vi "NI XNET CAN Signal Logger - Executor.vi"(8 "error in (no error)":errorcluster, 11 "Executor Command":refnum<user-event>) -> (0 "error out":errorcluster)   [LabVIEW 2021, in "XNET-CAN-Signal-Logger.lvlib"]
uses:
  XNET-CAN-Signal-Logger.lvlib
  Typedef/Def-Executor Command.ctl
  Def-ExecutorConfigurations.ctl
  Typedef/Def-LogSpec.ctl
  Typedef/Def-CAN Port Configuration.ctl
  Typedef/Def-Data Queue Ref.ctl
  Typedef/Def-Data Queue Type.ctl
  <userlib>/_NEVSTOP/NEVSTOP_TimerEngine/_Typedef/Timer-UserEvent.ctl
  Typedef/Def-GSTOP.ctl
  SubVIs/Global Variables.vi
  <userlib>/_NEVSTOP/GlobalStop/_gStop.vi
  <userlib>/_NEVSTOP/GlobalStop/GSTOP.lvlib
  <userlib>/_NEVSTOP/NEVSTOP_TimerEngine/TimerEngine.lvclass
panel:
  out "Monitor.Values":variant[](array[variant])
  out "Monitor.Names":variant[](array[variant])
  out "Signal Data":waveform(dbl)[](array[waveform])
  out "Signal Names":string[](array[string])
  out "Debug.WriterState":bool
  out "Debug.ReadersState":bool[](array[boolean])
  out "State":string="Preview..." caption="State:"
  out "# elements in queue":i32 caption="# elements in queue:"
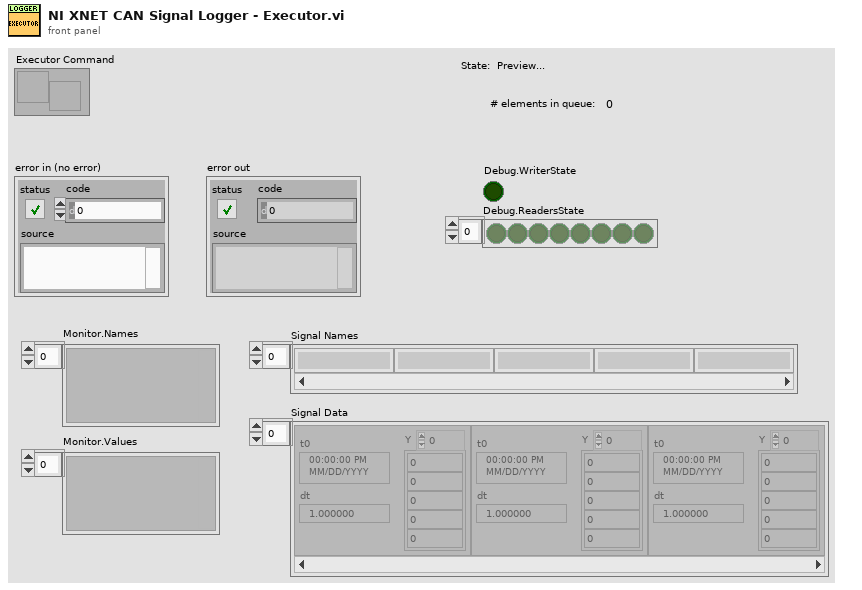
[diagram p1: front panel]
types:
  T1 = typedef "XNET-CAN-Signal-Logger.lvlib/Def-ExecutorConfigurations.ctl" = cluster{"LogSpec":T2, "CAN Configurations":T3[]}
  T2 = typedef "XNET-CAN-Signal-Logger.lvlib/Def-LogSpec.ctl" = cluster{"Log file folder":path, "Log file name":string, "Segment Files":bool, "Segment File Size":i64}
  T3 = typedef "XNET-CAN-Signal-Logger.lvlib/Def-CAN Port Configuration.ctl" = cluster{"CAN Interface":refnum<k21>, "XNET Cluster":refnum<k21>, "#Signals":i32, "Sample Rate (Hz)":dbl}
  T4 = enum32{"Invalid", "Standard", "Closed", "Hidden", "Minimized", "Maximized"}
  T5 = enum32{"invalid app kind", "Development System", "Run Time System", "Student Edition", "Embedded LabVIEW", "Evaluation", "Custom"}
  T6 = typedef "XNET-CAN-Signal-Logger.lvlib/Def-Executor Command.ctl" = cluster{"Command":string, "Data":variant}
  T7 = typedef "XNET-CAN-Signal-Logger.lvlib/Def-Data Queue Type.ctl" = cluster{"PackageID":i32, "Data":waveform(dbl)[]}
  T8 = typedef "XNET-CAN-Signal-Logger.lvlib/Def-GSTOP.ctl" = enum16{"Writer", "Readers"}
  T9 = typedef "XNET-CAN-Signal-Logger.lvlib/Def-Data Queue Ref.ctl" = refnum<queue>
  T10 = cluster{"Core":cluster{"Current VI Reference":refnum<vi>, "Close Panel on Exit?":bool}, "LogSpec":T2, "LogFilePath":path, "LogTS":timestamp, "CAN Configurations":T3[], "Signals to Monitor":string[][], "Data Queue Ref":T9, "Error Queue Ref":refnum<queue>, "State":string, "Executor Command":refnum<user-event>}
  T11 = cluster{"Current VI Reference":refnum<vi>, "Close Panel on Exit?":bool}
  T12 = typedef "TimerEngine.lvlib/TimerEngine.lvclass/Timer-UserEvent.ctl" = refnum<user-event>
  T13 = typedef "TimerEngine.lvlib/TimerEngine.lvclass/Timer-Userevent.ctl" = refnum<user-event>
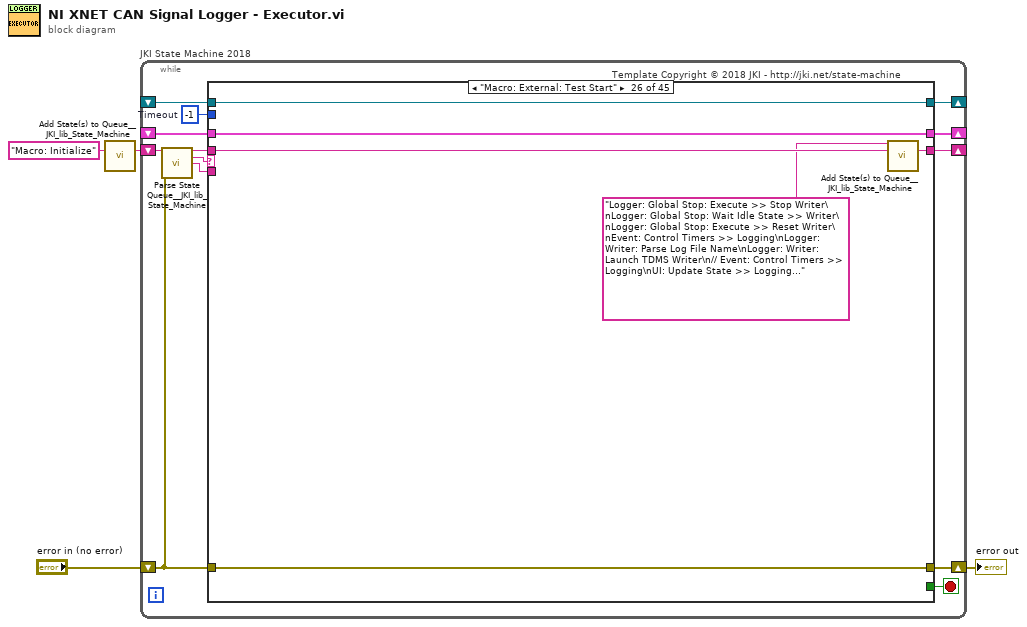
[diagram p0: block diagram]
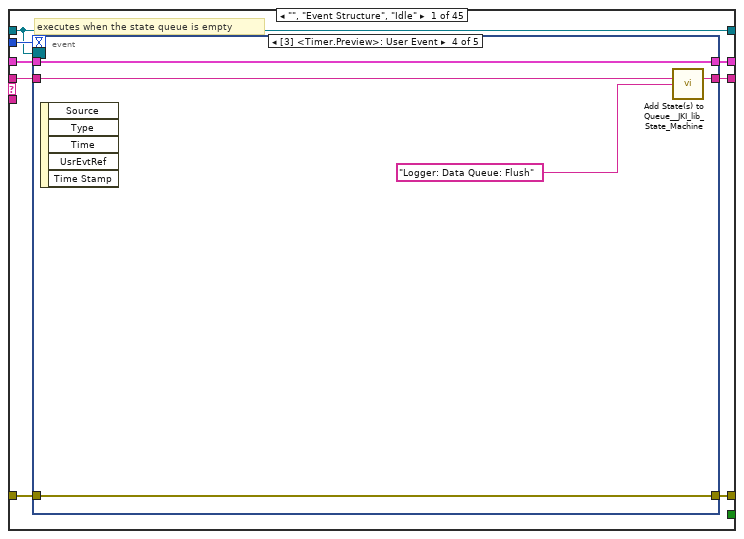
[diagram p2: hidden frame]
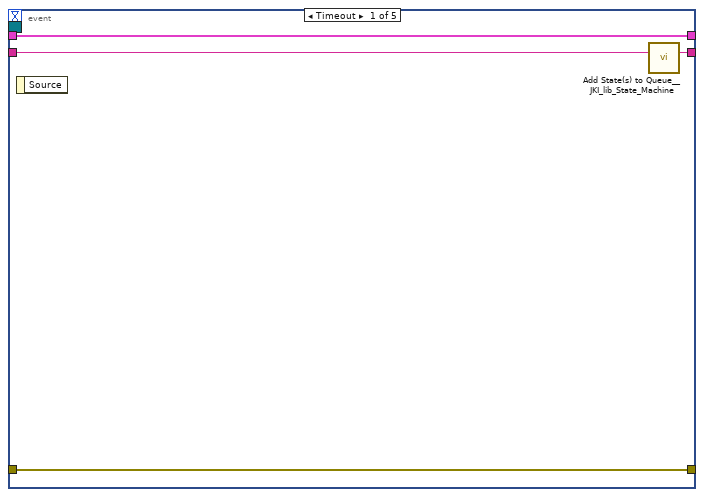
[diagram p3: hidden frame]
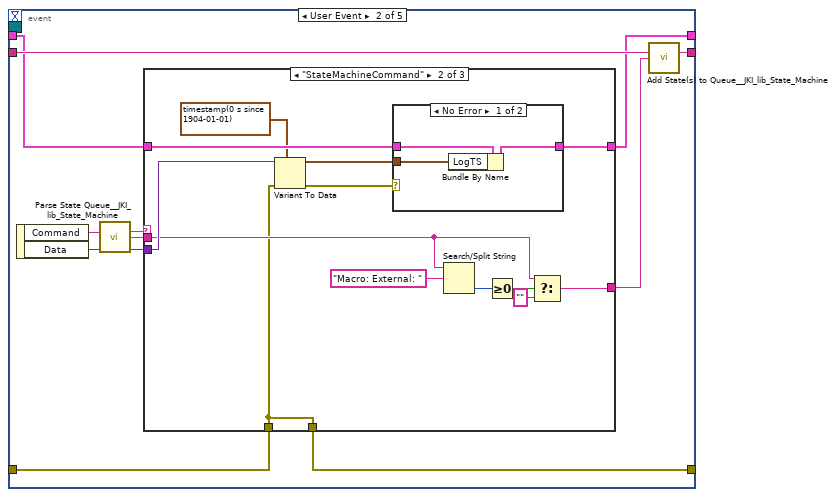
[diagram p4: hidden frame]
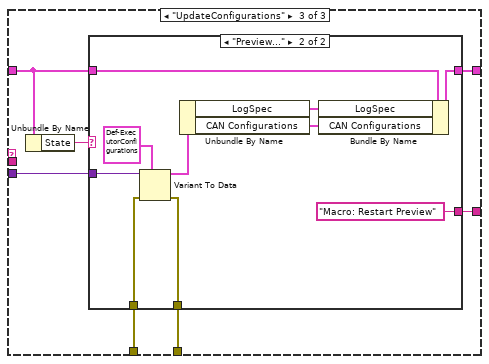
[diagram p7: hidden frame]
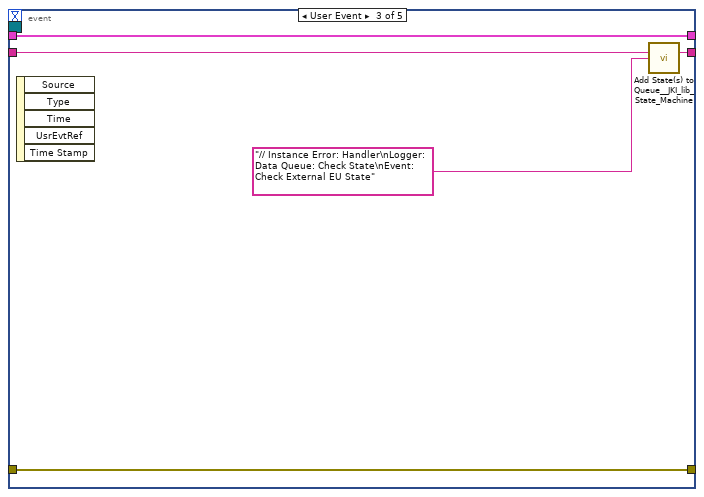
[diagram p9: hidden frame]
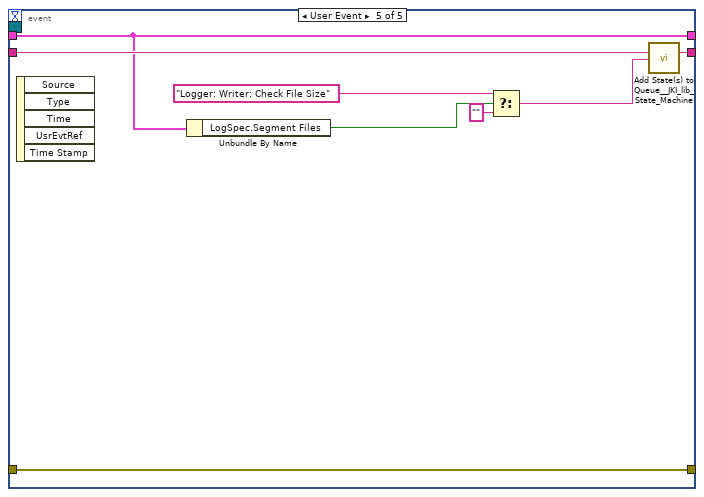
[diagram p10: hidden frame]
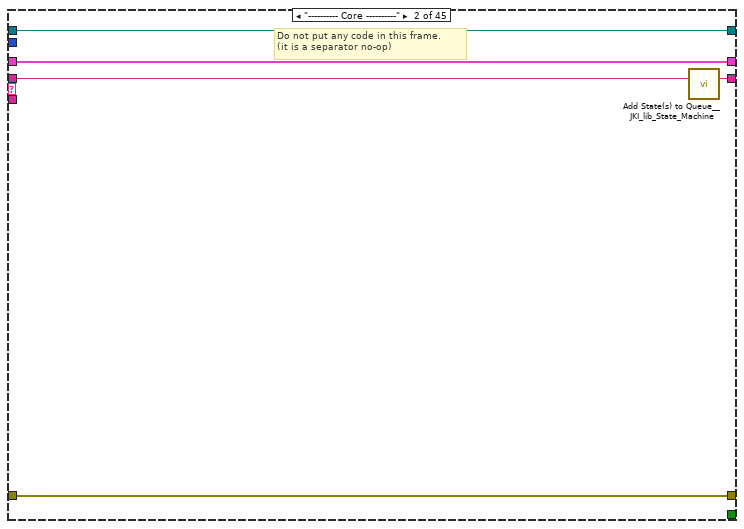
[diagram p11: hidden frame]
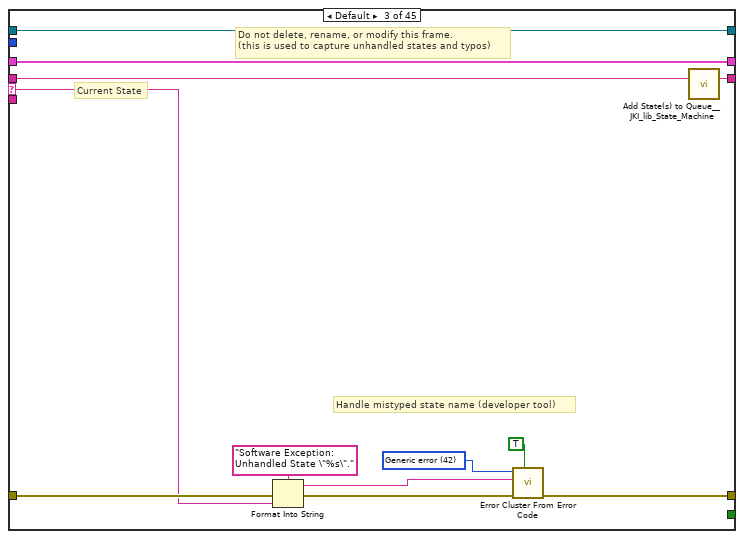
[diagram p12: hidden frame]
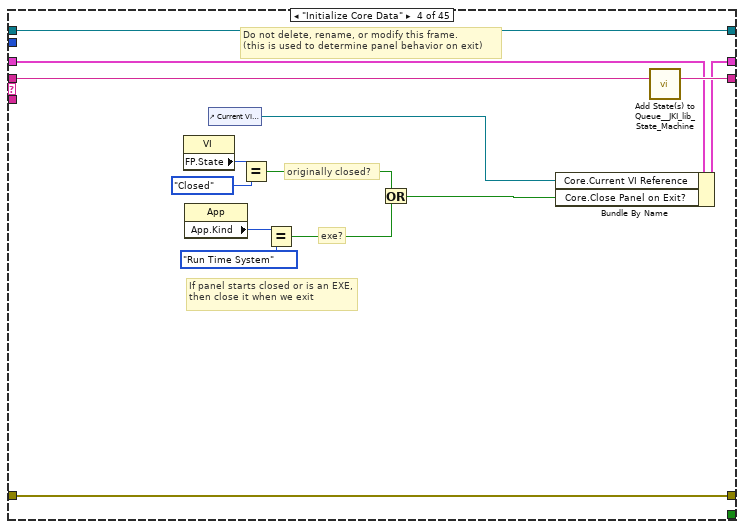
[diagram p13: hidden frame]
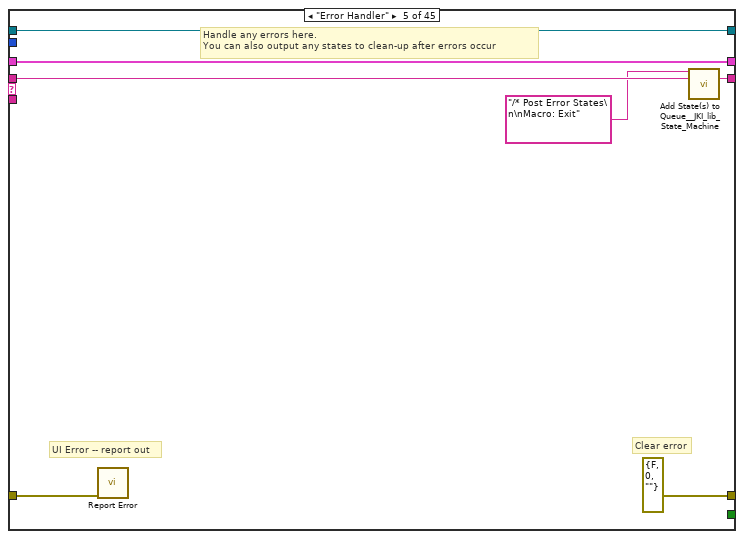
[diagram p14: hidden frame]
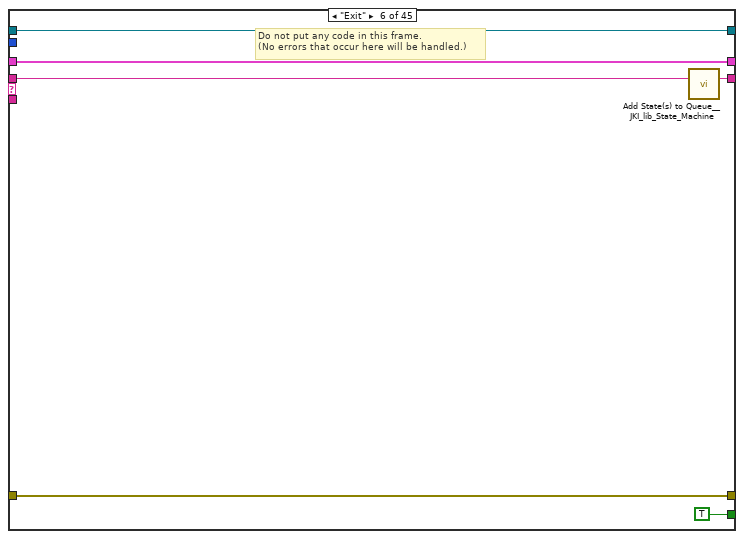
[diagram p15: hidden frame]
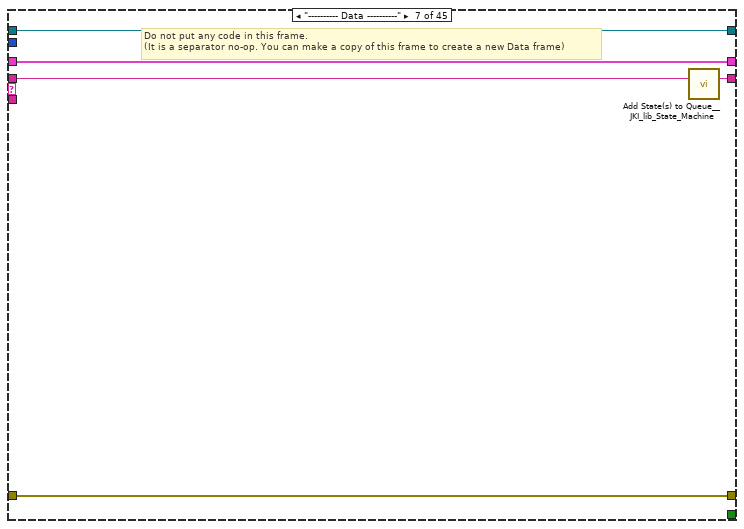
[diagram p16: hidden frame]
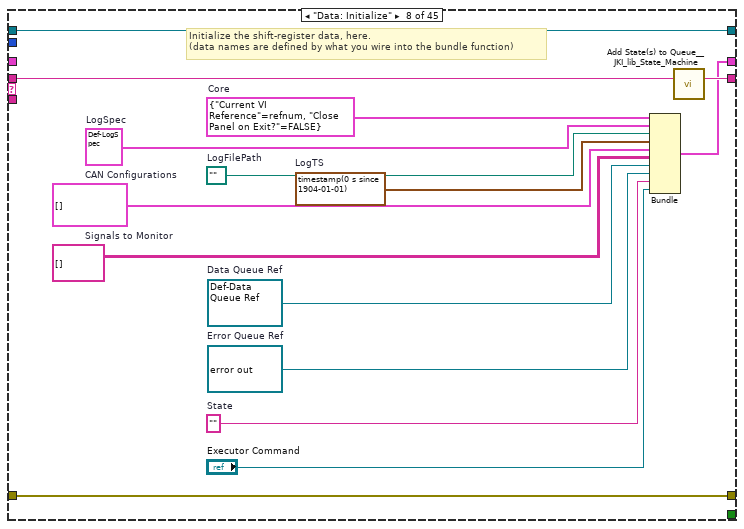
[diagram p17: hidden frame]
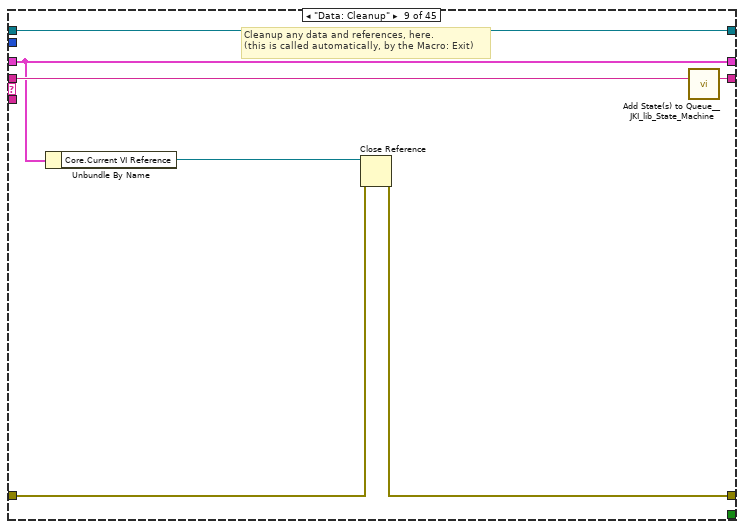
[diagram p18: hidden frame]
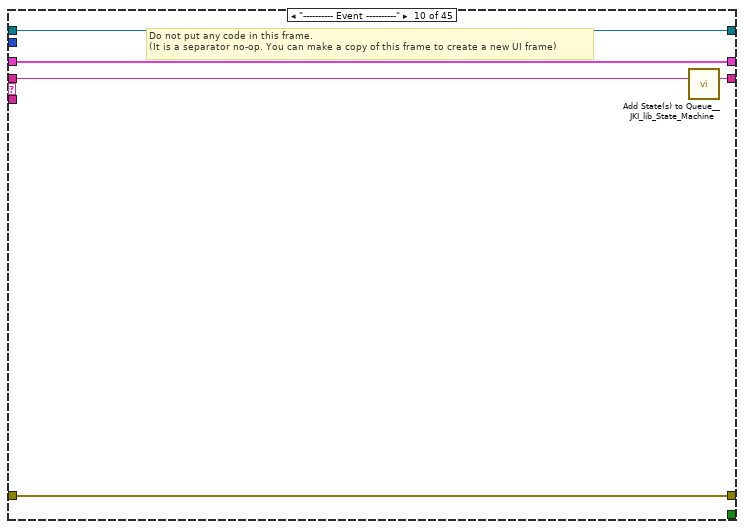
[diagram p19: hidden frame]
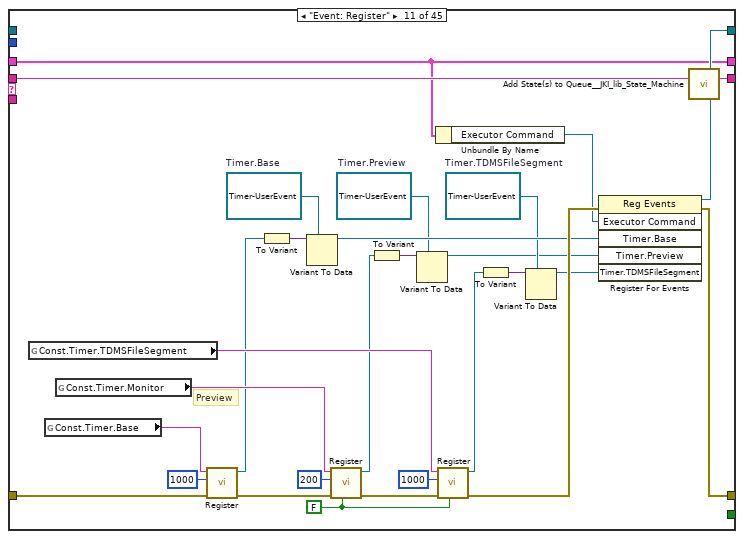
[diagram p20: hidden frame]
diagram:
  n1 = call <vilib>:"Add State(s) to Queue__JKI_lib_State_Machine.vi"("State(s) in (\"\")"="Macro: Initialize") -> ("States Out"=w4:string)  [unwired: 14 in]
  n2 = while "JKI State Machine 2018" {
    shift-right: [w10] -> _
    shift-left: _ -> [w9]
    shift-right: [w13] -> w1
    shift-left: "error in (no error)" -> [w7]
    shift-right: [w12] -> _
    shift-left: w4 -> [w14]
    shift-right: [w6] -> _
    shift-left: _ -> [w5]
    stop <- w11 stop-if-true
    w8 = -1  # Timeout
    # "Template Copyright © 2018 JKI - http://jki.net/state-machine"
    n3 = call <vilib>:"Parse State Queue__JKI_lib_State_Machine.vi"("State Queue"=w14, "Error In (no error)"=w7) -> ("Remaining States"=w16:string, "Current State"=w17:string, "Arguments"=w15:string)  [unwired: 11 in]
    n4 = case shown="\"Macro: External: Test Start\"" w17 {
      selector: w17 -> [_ _ w103 _ _ _ _ _ _ _ _ _ _ _ _ _ _ _ _ _ _ _ _ _ _ _ _ _ _ _ _ _ _ _ _ _ _ _ _ _ _ _ _ _ _]
      tunnel: w16 -> [w25 w101 w107 w127 w134 w140 w145 w160 w167 w172 w201 w210 w225 w240 w245 w253 w260 w272 w344 w349 w355 w361 w367 w373 w384 w390 w396 w402 w407 w417 w427 w438 w452 w457 w468 w477 w486 w502 w509 w516 w543 w555 w564 w571 w580]
      tunnel: w15 -> [_ _ _ _ _ _ _ _ _ _ _ _ w217 _ _ _ w255 w266 w338 _ _ _ _ _ _ _ _ _ _ _ _ _ _ _ _ _ _ _ _ w513 w536 _ _ _ _]
      tunnel: w9 -> [w23 w98 w105 w120 w131 w138 w142 _ w162 w169 w173 w208 w223 w236 w242 w251 w258 w268 w341 w346 w352 w358 w364 w370 w381 w387 w393 w399 w404 w415 w425 w436 w447 w454 w461 w475 w484 w500 w504 w514 w540 w552 w562 w569 w578]
      tunnel: [w22 w99 w109 w124 errorcluster {"status"=FALSE, "code"=0, "source"=""} ("error out") w137 w143 w157 w163 w170 w198 w202 w215 w238 w243 w250 w256 w269 w342 w347 w353 w359 w365 w371 w382 w388 w394 w400 w405 w411 w422 w433 w448 w455 w466 w473 w481 w489 w506 w511 w538 w553 w560 w566 w575] -> w13
      tunnel: w7 -> [w21 w99 w108 w124 w130 w137 w143 w157 w164 w170 w188 w206 w219 w238 w243 w250 w257 w270 w342 w347 w353 w359 w365 w371 w382 w388 w394 w400 w405 w412 w423 w434 w450 w455 w466 w470 w482 w498 w507 w512 w541 w553 w556 w567 w576]
      tunnel: [w24 w100 w106 w126 w133 w139 w144 w159 w166 w171 w200 w209 w224 w239 w244 w252 w259 w271 w343 w348 w354 w360 w366 w372 w383 w389 w395 w401 w406 w416 w426 w437 w451 w456 w467 w476 w485 w501 w508 w515 w542 w554 w563 w570 w579] -> w12
      tunnel: [_ _ _ _ _ TRUE _ _ _ _ _ _ _ _ _ _ _ _ _ _ _ _ _ _ _ _ _ _ _ _ _ _ _ _ _ _ _ _ _ _ _ _ _ _ _] -> w11
      tunnel: [w20 w98 w105 w125 w131 w138 w142 w158 w162 w169 w173 w208 w223 w236 w242 w251 w258 w268 w339 w346 w352 w358 w364 w370 w381 w387 w393 w399 w404 w410 w425 w436 w447 w454 w464 w475 w484 w500 w504 w514 w540 w552 w559 w569 w578] -> w10
      tunnel: w8 -> [w19 _ _ _ _ _ _ _ _ _ _ _ _ _ _ _ _ _ _ _ _ _ _ _ _ _ _ _ _ _ _ _ _ _ _ _ _ _ _ _ _ _ _ _ _]
      tunnel: [w18 w97 w102 w114 w128 w135 w141 w152 w161 w168 w199 w207 w218 w237 w241 w248 w254 w265 w340 w345 w350 w356 w363 w368 w374 w385 w391 w397 w403 w408 w420 w432 w449 w453 w462 w472 w480 w494 w505 w510 w539 w551 w557 w565 w574] -> w6
      tunnel: w5 -> [w18 w97 w102 w114 w128 w135 w141 w152 w161 w168 _ w207 w218 w237 w241 w248 w254 w265 w340 w345 w350 w356 w363 w368 w374 w385 w391 w397 w403 w408 w420 w432 w449 w453 w462 w472 w480 w494 w505 w510 w539 w551 w557 w565 w574]
      frame "", "Event Structure", "Idle" {
        # "executes when the state queue is empty"
        n5 = event shown="[3] <Timer.Preview>: User Event" {
          selector: w18 -> [_ _ _ _ _]
          dyn-events: _ -> [_ _ _ _ _]
          timeout: w19 -> [_ _ _ _ _]
          tunnel: w25 -> [w26 w39 w79 w85 w91]
          tunnel: [w29 w40 w83 w88 w96] -> w24
          tunnel: w23 -> [w27 w37 w81 w86 w90]
          tunnel: [w28 w32 w82 w87 w95] -> w22
          tunnel: w21 -> [w28 w33 w82 w87 w95]
          tunnel: [w27 w36 w81 w86 w90] -> w20
          event Timeout {
            n6 = event-data() -> ()  [unwired: 1 in, 1 out]
            n7 = call <vilib>:"Add State(s) to Queue__JKI_lib_State_Machine.vi"("State(s) in (\"\")"=w26) -> ("States Out"=w29:string)  [unwired: 14 in]
          }
          event User Event {
            n8 = event-data() -> ("Command"=w38:string, "Data"=w34:variant)  [unwired: 1 in]
            n9 = call <vilib>:"Parse State Queue__JKI_lib_State_Machine.vi"("State Queue"=w38) -> ("Current State"=w31:string, "Arguments"=w30:string)  [unwired: 12 in, 1 out]
            n10 = case shown="\"StateMachineCommand\"" w31 {
              tunnel: w37 -> [w42 w55 w63]
              tunnel: [w42 w46 w62] -> w36
              tunnel: [_ w49 w61] -> w35
              tunnel: w34 -> [_ w54 w66]
              tunnel: w33 -> [w41 w44 w65]
              tunnel: [w41 w44 w64] -> w32
              tunnel: w30 -> [_ w48 _]
              frame Default {
              }
              frame "StateMachineCommand" {
                n11 = Variant To Data(error in=w44, type=timestamp(0 s since 1904-01-01) ("Time Stamp"), Variant=w54) -> (data=w45:timestamp, error out=w43:errorcluster)
                n12 = case shown="No Error" w43 {
                  tunnel: w55 -> [w58 w59]
                  tunnel: [w57 w59] -> w46
                  tunnel: w45 -> [w56 _]
                  frame No Error {
                    n13 = Bundle By Name(cluster=w58, "LogTS"=w56) -> (w57:T10)
                  }
                  frame Error {
                  }
                }
                n14 = Search/Split String(string=w48, search string/char (-)="Macro: External: ") -> (offset of match=w52:i32)  [unwired: 1 in, 2 out]
                n15 = Greater Or Equal To 0?(x=w52) -> (x >= 0?=w51:bool)
                n16 = Select(t=w48, s=w51, f="") -> (s? t:f=w49:string)
              }
              frame "UpdateConfigurations" {
                n17 = Unbundle By Name(w63) -> ("State"=w60:string)
                n18 = case shown="\"Preview...\"" w60 {
                  tunnel: w66 -> [_ w78]
                  tunnel: w65 -> [w67 w77]
                  tunnel: [w67 w76] -> w64
                  tunnel: w63 -> [w68 w75]
                  tunnel: [w68 w74] -> w62
                  tunnel: [_ "Macro: Restart Preview" ("f")] -> w61
                  frame "False", Default {
                  }
                  frame "Preview..." {
                    n19 = Variant To Data(error in=w77, type=T1 {"LogSpec"={"Log file folder"=path "C:/Users/NI/Desktop/Data", "Log file name"="Plugin_LogFile_{Year}-{Month}-{Day}-{Hour}-{Minute}-{Second}.tdms", "Segment Files"=FALSE, "Segment File Size"=100}, "CAN Configurations"=[]} ("Executor Configurations"), Variant=w78) -> (data=w73:T1, error out=w76:errorcluster)
                    n20 = Unbundle By Name(w73) -> ("LogSpec"=w71:T2, "CAN Configurations"=w72:T3[])
                    n21 = Bundle By Name(cluster=w75, "LogSpec"=w71, "CAN Configurations"=w72) -> (w74:T10)
                  }
                }
              }
            }
            n22 = call <vilib>:"Add State(s) to Queue__JKI_lib_State_Machine.vi"("State(s) in (\"\")"=w39, "State(s) at Back (\"\")"=w35) -> ("States Out"=w40:string)  [unwired: 13 in]
          }
          event User Event {
            n23 = event-data() -> ()  [unwired: 1 in, 5 out]
            n24 = call <vilib>:"Add State(s) to Queue__JKI_lib_State_Machine.vi"("State(s) in (\"\")"=w79, "State(s) at Back (\"\")"="// Instance Error: Handler\nLogger: Data Queue: Check State\nEvent: Check External EU State" ("State(s) at Back (\"\")")) -> ("States Out"=w83:string)  [unwired: 13 in]
          }
          event User Event {
            n25 = event-data() -> ()  [unwired: 1 in, 5 out]
            n26 = call <vilib>:"Add State(s) to Queue__JKI_lib_State_Machine.vi"("State(s) in (\"\")"=w85, "State(s) at Back (\"\")"="Logger: Data Queue: Flush" ("State(s) at Back (\"\")")) -> ("States Out"=w88:string)  [unwired: 13 in]
          }
          event User Event {
            n27 = event-data() -> ()  [unwired: 1 in, 5 out]
            n28 = Unbundle By Name(w90) -> ("LogSpec.Segment Files"=w89:bool)
            n29 = Select(t="Logger: Writer: Check File Size" ("State(s) at Back (\"\")"), s=w89, f="") -> (s? t:f=w93:string)
            n30 = call <vilib>:"Add State(s) to Queue__JKI_lib_State_Machine.vi"("State(s) in (\"\")"=w91, "State(s) at Back (\"\")"=w93) -> ("States Out"=w96:string)  [unwired: 13 in]
          }
        }
      }
      frame "---------- Core ----------" {
        # "Do not put any code in this frame.\n(it is a separator no-op)"
        n31 = call <vilib>:"Add State(s) to Queue__JKI_lib_State_Machine.vi"("State(s) in (\"\")"=w101) -> ("States Out"=w100:string)  [unwired: 14 in]
      }
      frame Default {
        w112 = 42 items=["No error", "Argument error", "Memory is full", "Out of zone", "End of file", "File already open", "Generic file I/O error", "File not found", "File permission error", "Disk is full", "Duplicate path", "Too many files open", "System feature not enabled", "Resource file not found", "Cannot add resource", "Resource not found", "Image not found", "Image memory error", "Pen does not exist", "Config type invalid", "Config token not found", "Config parse error", "Config memory error", "Bad external code format", "Bad external code offset", "External code not present", "Null window", "Destroy window error", "Null menu", "Print aborted", "Bad print record", "Print driver error", "Windows error during printing", "Memory error during printing", "Print dialog error", "Generic print error", "Invalid device refnum", "Device not found", "Device parameter error", "Device unit error", "Cannot open device", "Device call aborted", "Generic error", "Cancelled by user", "Object ID too low", "Object ID too high", "Object not in heap", "Unknown heap", "Unknown object (invalid DefProc)", "Unknown object (DefProc not in table)", "Message out of range", "Invalid (null) method", "Unknown message", "Manager call not supported", "Bad address", "Network operation in progress", "Network operation timed out", "Connection is busy", "Network attribute not supported", "Network error", "Address in use", "System out of memory", "Connection aborted", "Connection refused", "Not connected", "Already connected", "Connection closed", "Initialization error (interapplication manager)", "Bad occurrence", "Wait on unbound occurrence handler", "Occurrence queue overflow", "Datalog type conflict", "Unused", "Unrecognized type (interapplication manager)", "Memory corrupt", "Failed to make temporary DLL", "Old CIN version", "Drag socket not found", "Failed to load drop-object", "Failed to register OLE object", "Failed to release OLE object", "Format specifier type mismatch", "Unknown format specifier", "Too few format specifiers", "Too many format specifiers", "Scan failed", "Newer CIN version", "Error converting to variant", "Runtime menu error", "Password tampered", "Variant attribute not found", "Incompatible variant data type", "Event data is not available", "Event Store is not present", "Occurrence is not found", "Event Queue is not created", "Event info is not available", "Refnum passed is NULL", "Error retrieving Class GUID", "Error retrieving CoClass GUID", "Error retrieving TypeLib GUID.", "Bad built application magic bytes.", "Specific driver is different from the specific driver associated with the Logical Name.", "There is no session opened to the class driver.", "Max Error", "MAX - Error with config objects", "MAX - Error loading configuration", "MAX - Group not supported"]
        # "Current State"
        # "Do not delete, rename, or modify this frame.\n(this is used to capture unhandled states and typos)"
        # "Handle mistyped state name (developer tool)"
        n32 = Format Into String(format string="Software Exception: Unhandled State \"%s\"." ("message"), error in=w108, w103) -> (resulting string=w111:string, error out=w110:errorcluster)  [unwired: 1 in]
        n33 = call <vilib>:"Error Cluster From Error Code.vi"("show call chain? (False)"=TRUE, "error in (no error)"=w110, "error message (\"\")"=w111, "error code (0)"=w112) -> ("error out"=w109:errorcluster)  [unwired: 5 in]
        n34 = call <vilib>:"Add State(s) to Queue__JKI_lib_State_Machine.vi"("State(s) in (\"\")"=w107) -> ("States Out"=w106:string)  [unwired: 14 in]
      }
      frame "Initialize Core Data" {
        # "Do not delete, rename, or modify this frame.\n(this is used to determine panel behavior on exit)"
        # "originally closed?"
        # "exe?"
        # "If panel starts closed or is an EXE, then close it when we exit"
        n35 = property class="VI"() -> ("FP.State"=w117:T4)  [unwired: 2 in, 2 out]
        n36 = property class="App"() -> ("App.Kind"=w123:T5)  [unwired: 2 in, 2 out]
        n37 = control-ref of="Current VI Reference"() -> (w118:refnum<vi>)
        n38 = Equal?(x=w117, y=T4."Closed" ("Front Panel Window:State")) -> (x = y?=w115:bool)
        n39 = Equal?(x=w123, y=T5."Run Time System" ("Application:Kind")) -> (x = y?=w121:bool)
        n40 = Or(x=w115, y=w121) -> (x .or. y?=w119:bool)
        n41 = Bundle By Name(cluster=w120, "Core.Current VI Reference"=w118, "Core.Close Panel on Exit?"=w119) -> (w125:T10)
        n42 = call <vilib>:"Add State(s) to Queue__JKI_lib_State_Machine.vi"("State(s) in (\"\")"=w127) -> ("States Out"=w126:string)  [unwired: 14 in]
      }
      frame "Error Handler" {
        # "UI Error -- report out"
        # "Handle any errors here.\nYou can also output any states to clean-up after errors occur"
        # "Clear error"
        n43 = call "Report Error.vi"("error in (no error)"=w130) -> ()  [unwired: 10 in, 1 out]
        n44 = call <vilib>:"Add State(s) to Queue__JKI_lib_State_Machine.vi"("State(s) in Front (\"\")"="/* Post Error States\n\nMacro: Exit", "State(s) in (\"\")"=w134) -> ("States Out"=w133:string)  [unwired: 13 in]
      }
      frame "Exit" {
        # "Do not put any code in this frame.\n(No errors that occur here will be handled.)"
        n45 = call <vilib>:"Add State(s) to Queue__JKI_lib_State_Machine.vi"("State(s) in (\"\")"=w140) -> ("States Out"=w139:string)  [unwired: 14 in]
      }
      frame "---------- Data ----------" {
        # "Do not put any code in this frame.\n(It is a separator no-op. You can make a copy of this frame to create a new Data frame)"
        n46 = call <vilib>:"Add State(s) to Queue__JKI_lib_State_Machine.vi"("State(s) in (\"\")"=w145) -> ("States Out"=w144:string)  [unwired: 14 in]
      }
      frame "Data: Initialize" {
        w147 = timestamp(0 s since 1904-01-01)  # LogTS
        w148 = ""  # State
        w149 = string[][] []  # Signals to Monitor
        w151 = T2 {"Log file folder"=path "C:/Users/NI/Desktop/Data", "Log file name"="Plugin_LogFile_{Year}-{Month}-{Day}-{Hour}-{Minute}-{Second}.tdms", "Segment Files"=FALSE, "Segment File Size"=100}  # LogSpec
        w150 = T3[] []  # CAN Configurations
        w153 = refnum<queue> refnum  # Error Queue Ref
        w154 = T9 refnum  # Data Queue Ref
        w155 = path ""  # LogFilePath
        w156 = T11 {"Current VI Reference"=refnum, "Close Panel on Exit?"=FALSE}  # Core
        # "Initialize the shift-register data, here.\n(data names are defined by what you wire into the bundle function)"
        n47 = Bundle("Core"=w156, "LogSpec"=w151, "LogFilePath"=w155, "LogTS"=w147, "CAN Configurations"=w150, "Signals to Monitor"=w149, "Data Queue Ref"=w154, "Error Queue Ref"=w153, "State"=w148, "Executor Command"="Executor Command") -> (w158:T10)  [unwired: 1 in]
        n48 = call <vilib>:"Add State(s) to Queue__JKI_lib_State_Machine.vi"("State(s) in (\"\")"=w160) -> ("States Out"=w159:string)  [unwired: 14 in]
      }
      frame "Data: Cleanup" {
        # "Cleanup any data and references, here.\n(this is called automatically, by the Macro: Exit)"
        n49 = Unbundle By Name(w162) -> ("Core.Current VI Reference"=w165:refnum<vi>)
        n50 = Close Reference(reference=w165, error in (no error)=w164) -> (error out=w163:errorcluster)
        n51 = call <vilib>:"Add State(s) to Queue__JKI_lib_State_Machine.vi"("State(s) in (\"\")"=w167) -> ("States Out"=w166:string)  [unwired: 14 in]
      }
      frame "---------- Event ----------" {
        # "Do not put any code in this frame.\n(It is a separator no-op. You can make a copy of this frame to create a new UI frame)"
        n52 = call <vilib>:"Add State(s) to Queue__JKI_lib_State_Machine.vi"("State(s) in (\"\")"=w172) -> ("States Out"=w171:string)  [unwired: 14 in]
      }
      frame "Event: Register" {
        w179 = T12 refnum  # Timer.TDMSFileSegment
        w182 = T12 refnum  # Timer.Preview
        w183 = T12 refnum  # Timer.Base
        w191 = FALSE ("Start Imidiatlely?(T)")
        # "Preview"
        n53 = global read "Global Variables.vi" "Const.Timer.TDMSFileSegment"() -> (w195:string)
        n54 = global read "Global Variables.vi" "Const.Timer.Base"() -> (w189:string)
        n55 = global read "Global Variables.vi" "Const.Timer.Monitor"() -> (w197:string)
        n56 = call <userlib>:"Register.vi"("error in (no error)"=w188, "TimePeroid(ms)"=1000, "Name"=w189) -> ("error out"=w187:errorcluster, "TimeupEvent"=w185:T13)  [unwired: 7 in]
        n57 = To Variant(anything=w185) -> (Variant=w186:variant)
        n58 = Variant To Data(type=w183, Variant=w186) -> (data=w184:T12)  [unwired: 1 in, 1 out]
        n59 = call <userlib>:"Register.vi"("Start Imidiatlely?(T)"=w191, "error in (no error)"=w187, "TimePeroid(ms)"=200, "Name"=w197) -> ("error out"=w196:errorcluster, "TimeupEvent"=w176:T13)  [unwired: 6 in]
        n60 = To Variant(anything=w176) -> (Variant=w181:variant)
        n61 = Variant To Data(type=w182, Variant=w181) -> (data=w175:T12)  [unwired: 1 in, 1 out]
        n62 = Unbundle By Name(w173) -> ("Executor Command"=w174:refnum<user-event>)
        n63 = call <userlib>:"Register.vi"("Start Imidiatlely?(T)"=w191, "error in (no error)"=w196, "TimePeroid(ms)"=1000, "Name"=w195) -> ("error out"=w192:errorcluster, "TimeupEvent"=w178:T13)  [unwired: 6 in]
        n64 = To Variant(anything=w178) -> (Variant=w180:variant)
        n65 = Variant To Data(type=w179, Variant=w180) -> (data=w177:T12)  [unwired: 1 in, 1 out]
        n66 = register-events(error in=w192, w174, w184, w175, w177) -> (reference out=w199:refnum<event-registration>, error out=w198:errorcluster)  [unwired: 1 in]
        n67 = call <vilib>:"Add State(s) to Queue__JKI_lib_State_Machine.vi"("State(s) in (\"\")"=w201) -> ("States Out"=w200:string)  [unwired: 14 in]
      }
      frame "Event: Unregister" {
        # "Do not put any code in this frame.\n(It is a separator no-op. You can make a copy of this frame to create a new UI frame)"
        n68 = Unregister For Events(event registration refnum=w207, error in=w206) -> (error out=w203:errorcluster)
        n69 = call <userlib>:"List Timers.vi"("error in (no error)"=w203) -> ("error out"=w205:errorcluster, "Timers"=w204:string[])  [unwired: 8 in, 1 out]
        n70 = for {
          tunnel: w204 -> [w212] mode=indexing
          shift-right: [w211] -> w202
          shift-left: w205 -> [w213]
          n71 = call <userlib>:"Unregister.vi"("error in (no error)"=w213, "Name"=w212) -> ("error out"=w211:errorcluster)  [unwired: 9 in]
        }
        n72 = call <vilib>:"Add State(s) to Queue__JKI_lib_State_Machine.vi"("State(s) in (\"\")"=w210) -> ("States Out"=w209:string)  [unwired: 14 in]
      }
      frame "Event: Control Timers" {
        # "Preview"
        n73 = case shown="\"Logging\", \"Start Logging\"" w217 {
          tunnel: [_ TRUE ("Start Imidiatlely?(T)") FALSE ("Start Imidiatlely?(T)")] -> w216
          tunnel: [_ FALSE ("Start Imidiatlely?(T)") TRUE ("Start Imidiatlely?(T)")] -> w214
          frame "Stop", "Stop All", Default {
          }
          frame "Preview", "Start Preview" {
          }
          frame "Logging", "Start Logging" {
          }
        }
        n74 = global read "Global Variables.vi" "Const.Timer.TDMSFileSegment"() -> (w220:string)
        n75 = global read "Global Variables.vi" "Const.Timer.Monitor"() -> (w222:string)
        n76 = call <userlib>:"Enable.vi"("error in (no error)"=w219, "Enable?"=w216, "Name"=w222) -> ("error out"=w221:errorcluster)  [unwired: 8 in]
        n77 = call <userlib>:"Enable.vi"("error in (no error)"=w221, "Enable?"=w214, "Name"=w220) -> ("error out"=w215:errorcluster)  [unwired: 8 in]
        n78 = call <vilib>:"Add State(s) to Queue__JKI_lib_State_Machine.vi"("State(s) in (\"\")"=w225) -> ("States Out"=w224:string)  [unwired: 14 in]
      }
      frame "Event: Check External EU State" {
        n79 = Unbundle By Name(w236) -> ("Executor Command"=w235:refnum<user-event>)
        n80 = Generate User Event(user event=w235, event data cluster=T6 {"Command"="", "Data"=variant} ("event data")) -> (error out=w233:errorcluster)  [unwired: 2 in, 1 out]
        n81 = Select(t="Macro: External: Exit" ("State(s) in Front (\"\")"), s=w233, f="") -> (s? t:f=w231:string)
        n82 = call <vilib>:"Add State(s) to Queue__JKI_lib_State_Machine.vi"("State(s) in Front (\"\")"=w231, "State(s) in (\"\")"=w240) -> ("States Out"=w239:string)  [unwired: 13 in]
      }
      frame "---------- UI ----------" {
        # "Do not put any code in this frame.\n(It is a separator no-op. You can make a copy of this frame to create a new UI frame)"
        n83 = call <vilib>:"Add State(s) to Queue__JKI_lib_State_Machine.vi"("State(s) in (\"\")"=w245) -> ("States Out"=w244:string)  [unwired: 14 in]
      }
      frame "UI: Initialize" {
        # "Initialize the User Interface, here.\n(this is called automatically, by the Macro: Init)"
        n84 = local write "# elements in queue"(0 ("# elements in queue:")) -> ()
        n85 = local write "State"("" ("State")) -> ()
        n86 = call <vilib>:"Add State(s) to Queue__JKI_lib_State_Machine.vi"("State(s) in Front (\"\")"="//UI: Front Panel State >> Open" ("State(s) in Front (\"\")"), "State(s) in (\"\")"=w253) -> ("States Out"=w252:string)  [unwired: 13 in]
      }
      frame "UI: Cursor Set" {
        # "Argument"
        # "Set and Unset Cursor Busy.\n(Usage: \"UI: Cursor Set >> Busy|Idle\")"
        n87 = case shown="\"Idle\", Default" w255 {
          tunnel: w257 -> [w262 w264]
          tunnel: [w261 w263] -> w256
          frame "Idle", Default {
            n88 = call <vilib>:"Unset Busy.vi"("error in (no error)"=w262) -> ("error out"=w261:errorcluster)  [unwired: 10 in]
          }
          frame "Busy" {
            n89 = call <vilib>:"Set Busy.vi"("error in (no error)"=w264) -> ("error out"=w263:errorcluster)  [unwired: 9 in, 1 out]
          }
        }
        n90 = call <vilib>:"Add State(s) to Queue__JKI_lib_State_Machine.vi"("State(s) in (\"\")"=w260) -> ("States Out"=w259:string)  [unwired: 14 in]
      }
      frame "UI: Front Panel State" {
        # "Argument"
        # "Set Front Panel Open or Closed\n(Usage: \"UI: Front Panel State >> Open|Close\")"
        n91 = Unbundle By Name(w268) -> ("Core.Current VI Reference"=w267:refnum<vi>)
        n92 = case shown="\"Minimize\", \"Minimized\"" w266 {
          tunnel: w270 -> [w278 w293 w304 w317 w330]
          tunnel: [w280 w294 w306 w319 w332] -> w269
          tunnel: w267 -> [w279 w291 w305 w318 w331]
          frame "Open", "Standard", Default {
            w273 = T4."Standard" ("State")
            n93 = property class="VI"(reference=w279, error in=w278) -> (reference out=w276:refnum<vi>, error out=w277:errorcluster, "FP.State"=w275:T4)
            n94 = Not Equal?(x=w275, y=w273) -> (x != y?=w274:bool)
            n95 = case shown="True" w274 {
              tunnel: [w284 w286] -> w280
              tunnel: w277 -> [w283 w286]
              tunnel: w276 -> [w282 _]
              tunnel: w273 -> [w281 _]
              frame True {
                n96 = invoke class="VI" method="FP.Open"(reference=w282, error in=w283, "Activate"=TRUE, "State"=w281) -> (error out=w284:errorcluster)  [unwired: 1 in, 4 out]
              }
              frame False {
              }
            }
          }
          frame "Close", "Closed" {
            n97 = property class="VI"(reference=w291, error in=w293) -> (reference out=w290:refnum<vi>, error out=w292:errorcluster, "FP.State"=w288:T4)
            n98 = Not Equal?(x=w288, y=T4."Closed" ("Front Panel Window:State")) -> (x != y?=w287:bool)
            n99 = case shown="True" w287 {
              tunnel: [w295 w298] -> w294
              tunnel: w292 -> [w295 w297]
              tunnel: w290 -> [_ w296]
              frame False {
              }
              frame True {
                n100 = invoke class="VI" method="FP.Close"(reference=w296, error in=w297) -> (error out=w298:errorcluster)  [unwired: 1 in, 2 out]
              }
            }
          }
          frame "Hidden", "Hide" {
            w299 = T4."Hidden" ("State")
            n101 = property class="VI"(reference=w305, error in=w304) -> (reference out=w302:refnum<vi>, error out=w303:errorcluster, "FP.State"=w301:T4)
            n102 = Not Equal?(x=w301, y=w299) -> (x != y?=w300:bool)
            n103 = case shown="True" w300 {
              tunnel: [w310 w311] -> w306
              tunnel: w303 -> [w309 w311]
              tunnel: w302 -> [w308 _]
              tunnel: w299 -> [w307 _]
              frame True {
                n104 = invoke class="VI" method="FP.Open"(reference=w308, error in=w309, "State"=w307) -> (error out=w310:errorcluster)  [unwired: 2 in, 4 out]
              }
              frame False {
              }
            }
          }
          frame "Minimize", "Minimized" {
            w312 = T4."Minimized" ("State")
            n105 = property class="VI"(reference=w318, error in=w317) -> (reference out=w315:refnum<vi>, error out=w316:errorcluster, "FP.State"=w314:T4)
            n106 = Not Equal?(x=w314, y=w312) -> (x != y?=w313:bool)
            n107 = case shown="True" w313 {
              tunnel: [w323 w324] -> w319
              tunnel: w316 -> [w322 w324]
              tunnel: w315 -> [w321 _]
              tunnel: w312 -> [w320 _]
              frame True {
                n108 = invoke class="VI" method="FP.Open"(reference=w321, error in=w322, "State"=w320) -> (error out=w323:errorcluster)  [unwired: 2 in, 4 out]
              }
              frame False {
              }
            }
          }
          frame "Maximize", "Maximized" {
            w325 = T4."Maximized" ("State")
            n109 = property class="VI"(reference=w331, error in=w330) -> (reference out=w328:refnum<vi>, error out=w329:errorcluster, "FP.State"=w327:T4)
            n110 = Not Equal?(x=w327, y=w325) -> (x != y?=w326:bool)
            n111 = case shown="True" w326 {
              tunnel: [w336 w337] -> w332
              tunnel: w329 -> [w335 w337]
              tunnel: w328 -> [w334 _]
              tunnel: w325 -> [w333 _]
              frame True {
                n112 = invoke class="VI" method="FP.Open"(reference=w334, error in=w335, "State"=w333) -> (error out=w336:errorcluster)  [unwired: 2 in, 4 out]
              }
              frame False {
              }
            }
          }
        }
        n113 = call <vilib>:"Add State(s) to Queue__JKI_lib_State_Machine.vi"("State(s) in (\"\")"=w272) -> ("States Out"=w271:string)  [unwired: 14 in]
      }
      frame "UI: Update State" {
        n114 = Bundle By Name(cluster=w341, "State"=w338) -> (w339:T10)
        n115 = call <vilib>:"Add State(s) to Queue__JKI_lib_State_Machine.vi"("State(s) in (\"\")"=w344) -> ("States Out"=w343:string)  [unwired: 14 in]
        "State" <- w338
      }
      frame "---------- Macro ----------" {
        # "Do not put any code in this frame.\n(It is a separator no-op. You can make a copy of this frame to create a new Macro frame)"
        n116 = call <vilib>:"Add State(s) to Queue__JKI_lib_State_Machine.vi"("State(s) in (\"\")"=w349) -> ("States Out"=w348:string)  [unwired: 14 in]
      }
      frame "Macro: Initialize" {
        # "Initialization Macro\n(This is called once, when the VI starts)"
        n117 = call <vilib>:"Add State(s) to Queue__JKI_lib_State_Machine.vi"("State(s) in Front (\"\")"="Data: Initialize\nInitialize Core Data\nEvent: Register\n// Instance Error: Obtain Error Queue\nUI: Initialize\n\nMacro: Start Preview", "State(s) in (\"\")"=w355) -> ("States Out"=w354:string)  [unwired: 13 in]
      }
      frame "Macro: Start Preview" {
        n118 = call <vilib>:"Add State(s) to Queue__JKI_lib_State_Machine.vi"("State(s) in Front (\"\")"="Logger: Data Queue: Obtain\nLogger: Global Stop: Execute >> Init\nLogger: Global Stop: Execute >> Stop\nLogger: Global Stop: Wait Idle State >> Readers\nLogger: Global Stop: Wait Idle State >> Writer\nLogger: Global Stop: Execute >> Reset\nLogger: Monitor: Initialize\nLogger: Readers: Launch XNET CAN Reader\nEvent: Control Timers >> Preview\nUI: Update State >> Preview..." ("State(s) in Front (\"\")"), "State(s) in (\"\")"=w361) -> ("States Out"=w360:string)  [unwired: 13 in]
      }
      frame "Macro: Restart Preview" {
        n119 = call <vilib>:"Add State(s) to Queue__JKI_lib_State_Machine.vi"("State(s) in Front (\"\")"="Logger: Global Stop: Execute >> Stop Readers\nLogger: Global Stop: Wait Idle State >> Readers\nLogger: Global Stop: Execute >> Reset Readers\nLogger: Monitor: Initialize\nLogger: Readers: Launch XNET CAN Reader" ("State(s) in Front (\"\")"), "State(s) in (\"\")"=w367) -> ("States Out"=w366:string)  [unwired: 13 in]
      }
      frame "Macro: Segment File" {
        n120 = call <vilib>:"Add State(s) to Queue__JKI_lib_State_Machine.vi"("State(s) in Front (\"\")"="Logger: Global Stop: Execute >> Stop Writer\nLogger: Global Stop: Wait Idle State >> Writer\nLogger: Global Stop: Execute >> Reset Writer\nLogger: Writer: Parse Log File Name\nLogger: Writer: Launch TDMS Writer Segmented" ("State(s) in Front (\"\")"), "State(s) in (\"\")"=w373) -> ("States Out"=w372:string)  [unwired: 13 in]
      }
      frame "Macro: Exit" {
        # "Exit Macro\n(This is called once, when the VI exits)"
        n121 = Unbundle By Name(w381) -> ("Core.Close Panel on Exit?"=w380:bool)
        n122 = Select(t="UI: Front Panel State >> Close", s=w380, f="") -> (s? t:f=w377:string)
        n123 = call <vilib>:"Add State(s) to Queue__JKI_lib_State_Machine.vi"("State(s) in (\"\")"=w377, "State(s) at Back (\"\")"="Logger: Global Stop: Execute >> Stop All\nEvent: Control Timers >> Stop All\n// Instance Error: Release Error Queue\n\nData: Cleanup\nEvent: Unregister\n\nExit") -> ("States Out"=w375:string)  [unwired: 13 in]
        n124 = call <vilib>:"Add State(s) to Queue__JKI_lib_State_Machine.vi"("State(s) in Front (\"\")"=w375, "State(s) in (\"\")"=w384) -> ("States Out"=w383:string)  [unwired: 13 in]
      }
      frame "Macro: External: Test Start" {
        n125 = call <vilib>:"Add State(s) to Queue__JKI_lib_State_Machine.vi"("State(s) in Front (\"\")"="Logger: Global Stop: Execute >> Stop Writer\nLogger: Global Stop: Wait Idle State >> Writer\nLogger: Global Stop: Execute >> Reset Writer\nEvent: Control Timers >> Logging\nLogger: Writer: Parse Log File Name\nLogger: Writer: Launch TDMS Writer\n// Event: Control Timers >> Logging\nUI: Update State >> Logging..." ("State(s) in Front (\"\")"), "State(s) in (\"\")"=w390) -> ("States Out"=w389:string)  [unwired: 13 in]
      }
      frame "Macro: External: Test Stop" {
        n126 = call <vilib>:"Add State(s) to Queue__JKI_lib_State_Machine.vi"("State(s) in Front (\"\")"="Logger: Global Stop: Execute >> Stop Writer\nLogger: Global Stop: Wait Idle State >> Writer\nLogger: Global Stop: Execute >> Reset Writer\nEvent: Control Timers >> Preview\nUI: Update State >> Preview..." ("State(s) in Front (\"\")"), "State(s) in (\"\")"=w396) -> ("States Out"=w395:string)  [unwired: 13 in]
      }
      frame "Macro: External: Exit" {
        n127 = call <vilib>:"Add State(s) to Queue__JKI_lib_State_Machine.vi"("State(s) in Front (\"\")"="Macro: Exit" ("State(s) in Front (\"\")"), "State(s) in (\"\")"=w402) -> ("States Out"=w401:string)  [unwired: 13 in]
      }
      frame "---------- Logger ----------" {
        # "Template Separator\n(You can make a copy of, or modify, this frame)"
        n128 = call <vilib>:"Add State(s) to Queue__JKI_lib_State_Machine.vi"("State(s) in (\"\")"=w407) -> ("States Out"=w406:string)  [unwired: 14 in]
      }
      frame "Logger: Data Queue: Obtain" {
        n129 = global read "Global Variables.vi" "Const.TDMSDataQueueName"() -> (w414:string)
        n130 = Obtain Queue(name (unnamed)=w414, element data type=T7 {"PackageID"=0, "Data"=[]} ("Data Queue Type"), error in (no error)=w412) -> (queue out=w409:refnum<queue>, error out=w411:errorcluster)  [unwired: 2 in, 1 out]
        n131 = Bundle By Name(cluster=w415, "Data Queue Ref"=w409) -> (w410:T10)
        n132 = call <vilib>:"Add State(s) to Queue__JKI_lib_State_Machine.vi"("State(s) in (\"\")"=w417) -> ("States Out"=w416:string)  [unwired: 14 in]
      }
      frame "Logger: Data Queue: Check State" {
        n133 = Unbundle By Name(w425) -> ("Data Queue Ref"=w424:T9)
        n134 = global read "Global Variables.vi" "Debug.ReadersState"() -> (→"Debug.ReadersState":bool[])
        n135 = global read "Global Variables.vi" "Debug.WriterState"() -> (→"Debug.WriterState":bool)
        n136 = Get Queue Status(queue=w424, error in (no error)=w423) -> (error out=w422:errorcluster, # elements in queue=→"# elements in queue":i32)  [unwired: 1 in, 6 out]
        n137 = call <vilib>:"Add State(s) to Queue__JKI_lib_State_Machine.vi"("State(s) in (\"\")"=w427) -> ("States Out"=w426:string)  [unwired: 14 in]
      }
      frame "Logger: Data Queue: Flush" {
        n138 = Unbundle By Name(w436) -> ("Data Queue Ref"=w435:T9)
        n139 = Flush Queue(queue=w435, error in (no error)=w434) -> (error out=w433:errorcluster)  [unwired: 2 out]
        n140 = global read "Global Variables.vi" "Monitor.Names"() -> (→"Monitor.Names":variant[])
        n141 = global read "Global Variables.vi" "Monitor.Values"() -> (→"Monitor.Values":variant[])
        n142 = call "Get Monitor.Names All.vi"() -> ("Signal Names"=→"Signal Names":string[])  [unwired: 10 in, 1 out]
        n143 = call "Get Monitor.Values All.vi"() -> ("Signal Data"=→"Signal Data":waveform(dbl)[])  [unwired: 10 in, 1 out]
        n144 = call <vilib>:"Add State(s) to Queue__JKI_lib_State_Machine.vi"("State(s) in (\"\")"=w438) -> ("States Out"=w437:string)  [unwired: 14 in]
      }
      frame "Logger: Monitor: Initialize" {
        # "Template Separator\n(You can make a copy of, or modify, this frame)"
        n145 = Unbundle By Name(w447) -> ("CAN Configurations"=w439:T3[])
        n146 = Array Size(array=w439) -> (size(s)=w443:i32)
        n147 = To Variant(anything=waveform(dbl)[] [] ("Data")) -> (Variant=w445:variant)
        n148 = Compound Arithmetic op=ADD(w443) -> (w441:i32)
        n149 = Initialize Array(w445, w441) -> (w444:variant[])
        n150 = Initialize Array(FALSE, w441) -> (w440:bool[])
        n151 = call "Query Signal Lists.vi"("error in (no error)"=w450, "CAN Configurations in"=w439) -> ("error out"=w448:errorcluster)  [unwired: 7 in, 2 out]
        n152 = global write "Global Variables.vi" "Monitor.Values"(w444) -> ()
        n153 = global write "Global Variables.vi" "Debug.ReadersState"(w440) -> ()
        n154 = call <vilib>:"Add State(s) to Queue__JKI_lib_State_Machine.vi"("State(s) in (\"\")"=w452) -> ("States Out"=w451:string)  [unwired: 14 in]
      }
      frame "Logger: Monitor: Update" {
        n155 = call <vilib>:"Add State(s) to Queue__JKI_lib_State_Machine.vi"("State(s) in (\"\")"=w457) -> ("States Out"=w456:string)  [unwired: 14 in]
      }
      frame "Logger: Writer: Parse Log File Name" {
        n156 = Unbundle By Name(w461) -> ("LogSpec.Log file folder"=w458:path, "LogTS"=w459:timestamp, "LogSpec.Log file name"=w460:string)
        n157 = call "Parse Log File Name.vi"("TimeStamp"=w459, "Log file name"=w460) -> ("Parsed Log file name"=w465:string)  [unwired: 9 in]
        n158 = Build Path(base path=w458, name or relative path=w465) -> (appended path=w463:path)
        n159 = Bundle By Name(cluster=w461, "LogFilePath"=w463) -> (w464:T10)
        n160 = call <vilib>:"Add State(s) to Queue__JKI_lib_State_Machine.vi"("State(s) in (\"\")"=w468) -> ("States Out"=w467:string)  [unwired: 14 in]
      }
      frame "Logger: Writer: Launch TDMS Writer" {
        n161 = Unbundle By Name(w475) -> ("LogTS"=w469:timestamp, "LogFilePath"=w474:path, "CAN Configurations"=w471:T3[])
        n162 = call "Launch Action - TDMS Writer.vi"("Time Stamp"=w469, "error in (no error)"=w470, "CAN Configurations"=w471, "Log file path"=w474) -> ("error out"=w473:errorcluster)  [unwired: 7 in]
        n163 = call <vilib>:"Add State(s) to Queue__JKI_lib_State_Machine.vi"("State(s) in (\"\")"=w477) -> ("States Out"=w476:string)  [unwired: 14 in]
      }
      frame "Logger: Writer: Launch TDMS Writer Segmented" {
        n164 = Unbundle By Name(w484) -> ("LogTS"=w478:timestamp, "LogFilePath"=w483:path, "CAN Configurations"=w479:T3[])
        n165 = call "Launch Action - TDMS Writer Segmented.vi"("Time Stamp"=w478, "error in (no error)"=w482, "CAN Configurations"=w479, "Log file path"=w483) -> ("error out"=w481:errorcluster)  [unwired: 7 in]
        n166 = call <vilib>:"Add State(s) to Queue__JKI_lib_State_Machine.vi"("State(s) in (\"\")"=w486) -> ("States Out"=w485:string)  [unwired: 14 in]
      }
      frame "Logger: Writer: Check File Size" {
        # "create new file to segment file"
        n167 = Unbundle By Name(w500) -> ("LogSpec.Segment File Size"=w487:i64, "LogFilePath"=w499:path)
        n168 = Get File Size(file=w499, error in=w498) -> (size (in bytes)=w496:i64, 0:w497:errorcluster)  [unwired: 1 out]
        n169 = Logical Shift(y=i16 -20, x=w496) -> (x << y=w490:i64)
        n170 = call <vilib>:"Clear Errors.vi"("error in (no error)"=w497) -> ("error out"=w489:errorcluster)  [unwired: 5 in, 1 out]
        n171 = Greater Or Equal?(x=w490, y=w487) -> (x >= y?=w492:bool)
        n172 = Select(t="Macro: Segment File" ("State(s) at Back (\"\")"), s=w492, f="") -> (s? t:f=w488:string)
        n173 = call <vilib>:"Add State(s) to Queue__JKI_lib_State_Machine.vi"("State(s) in Front (\"\")"=w488, "State(s) in (\"\")"=w502) -> ("States Out"=w501:string)  [unwired: 13 in]
      }
      frame "Logger: Readers: Launch XNET CAN Reader" {
        n174 = Unbundle By Name(w504) -> ("CAN Configurations"=w503:T3[])
        n175 = call "Launch Action - XNET CAN Readers.vi"("error in (no error)"=w507, "CAN Configurations"=w503) -> ("error out"=w506:errorcluster)  [unwired: 9 in]
        n176 = call <vilib>:"Add State(s) to Queue__JKI_lib_State_Machine.vi"("State(s) in (\"\")"=w509) -> ("States Out"=w508:string)  [unwired: 14 in]
      }
      frame "Logger: Global Stop: Execute" {
        # "Template Separator\n(You can make a copy of, or modify, this frame)"
        n177 = case shown="\"Reset Writer\"" w513 {
          tunnel: w512 -> [w517 w519 w521 w524 w527 w529 w532 w535]
          tunnel: [w517 w518 w520 w523 w526 w528 w531 w534] -> w511
          frame Default {
          }
          frame "Init" {
            n178 = call <userlib>:"GSTOP INIT.vi"("error in (no error)"=w519) -> ("error out"=w518:errorcluster)  [unwired: 14 in]
          }
          frame "Stop", "Stop All" {
            n179 = call <userlib>:"GSTOP SET.vi"("error in (no error)"=w521) -> ("error out"=w520:errorcluster)  [unwired: 14 in]
          }
          frame "Stop Writer" {
            n180 = call <userlib>:"GSTOP SET.vi"("index(-1 for All)"=Def-GSTOP."Writer" ("GSTOP"), "error in (no error)"=w524) -> ("error out"=w523:errorcluster)  [unwired: 13 in]
          }
          frame "Stop Readers" {
            n181 = call <userlib>:"GSTOP SET.vi"("index(-1 for All)"=Def-GSTOP."Readers" ("GSTOP"), "error in (no error)"=w527) -> ("error out"=w526:errorcluster)  [unwired: 13 in]
          }
          frame "Reset", "Reset All" {
            n182 = call <userlib>:"GSTOP RESET.vi"("error in (no error)"=w529) -> ("error out"=w528:errorcluster)  [unwired: 14 in]
          }
          frame "Reset Writer" {
            n183 = call <userlib>:"GSTOP RESET.vi"("index(-1 for All)"=Def-GSTOP."Writer" ("GSTOP"), "error in (no error)"=w532) -> ("error out"=w531:errorcluster)  [unwired: 13 in]
          }
          frame "Reset Readers" {
            n184 = call <userlib>:"GSTOP RESET.vi"("index(-1 for All)"=Def-GSTOP."Readers" ("GSTOP"), "error in (no error)"=w535) -> ("error out"=w534:errorcluster)  [unwired: 13 in]
          }
        }
        n185 = call <vilib>:"Add State(s) to Queue__JKI_lib_State_Machine.vi"("State(s) in (\"\")"=w516) -> ("States Out"=w515:string)  [unwired: 14 in]
      }
      frame "Logger: Global Stop: Wait Idle State" {
        w537 = FALSE  # Target WriterState (T-Running/F-Idle)
        # "Template Separator\n(You can make a copy of, or modify, this frame)"
        n186 = case shown="\"Readers\"" w536 {
          tunnel: w541 -> [w544 w547 w550]
          tunnel: [w544 w546 w549] -> w538
          tunnel: w537 -> [_ w545 w548]
          frame Default {
          }
          frame "Writer" {
            n187 = call "Wait for WriterState.vi"("error in (no error)"=w547, "Target WriterState (T-Running/F-Idle)"=w545) -> ("error out"=w546:errorcluster)  [unwired: 8 in, 1 out]
          }
          frame "Readers" {
            n188 = call "Wait for ReaderState.vi"("error in (no error)"=w550, "Target WriterState (T-Running/F-Idle)"=w548) -> ("error out"=w549:errorcluster)  [unwired: 8 in, 1 out]
          }
        }
        n189 = call <vilib>:"Add State(s) to Queue__JKI_lib_State_Machine.vi"("State(s) in (\"\")"=w543) -> ("States Out"=w542:string)  [unwired: 14 in]
      }
      frame "---------- Instance Error ----------" {
        # "Template Separator\n(You can make a copy of, or modify, this frame)"
        n190 = call <vilib>:"Add State(s) to Queue__JKI_lib_State_Machine.vi"("State(s) in (\"\")"=w555) -> ("States Out"=w554:string)  [unwired: 14 in]
      }
      frame "Instance Error: Obtain Error Queue" {
        n191 = global read "Global Variables.vi" "Const.ErrorQueueName"() -> (w561:string)
        n192 = Obtain Queue(name (unnamed)=w561, element data type=w556, error in (no error)=w556) -> (queue out=w558:refnum<queue>, error out=w560:errorcluster)  [unwired: 2 in, 1 out]
        n193 = Bundle By Name(cluster=w562, "Error Queue Ref"=w558) -> (w559:T10)
        n194 = call <vilib>:"Add State(s) to Queue__JKI_lib_State_Machine.vi"("State(s) in (\"\")"=w564) -> ("States Out"=w563:string)  [unwired: 14 in]
      }
      frame "Instance Error: Release Error Queue" {
        n195 = Unbundle By Name(w569) -> ("Error Queue Ref"=w568:refnum<queue>)
        n196 = Release Queue(queue=w568, error in (no error)=w567) -> (error out=w566:errorcluster)  [unwired: 1 in, 2 out]
        n197 = call <vilib>:"Add State(s) to Queue__JKI_lib_State_Machine.vi"("State(s) in (\"\")"=w571) -> ("States Out"=w570:string)  [unwired: 14 in]
      }
      frame "Instance Error: Handler" {
        # "Instance Error -- Display it"
        n198 = Unbundle By Name(w578) -> ("Error Queue Ref"=w577:refnum<queue>)
        n199 = Dequeue Element(queue=w577, timeout in ms (-1)=0, error in (no error)=w576) -> (element=w572:errorcluster, error out=w575:errorcluster)  [unwired: 2 out]
        n200 = call <vilib>:"General Error Handler.vi"("error in (no error)"=w572) -> ()  [unwired: 10 in, 5 out]
        n201 = call <vilib>:"Add State(s) to Queue__JKI_lib_State_Machine.vi"("State(s) in (\"\")"=w580) -> ("States Out"=w579:string)  [unwired: 14 in]
      }
    }
  }
  "error out" <- w1
